vi "Critical.vi"(8 "error in (no error)":errorcluster, 9 "Source":string, 10 "Message":string, 11 "RQMHLogger in":refnum<class "RQMHLogger.lvclass">) -> (0 "error out":errorcluster, 3 "RQMHLogger out":refnum<class "RQMHLogger.lvclass">)   [LabVIEW 2024, in "RQMHLogger.lvclass"]
uses:
  RQMHLogger.lvclass
  RQMHLogger.lvclass/RQMHLogger.ctl
  Shared/Level.ctl
  Shared/LoggerShared.lvlib
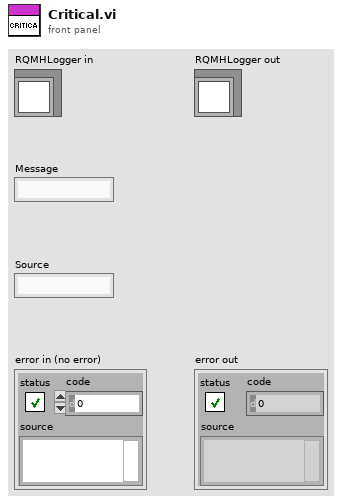
[diagram p1: front panel]
types:
  T1 = typedef "LoggerShared.lvlib/Level.ctl" = enum16{"DEBUG", "INFO", "WARNING", "ERROR", "CRITICAL"}
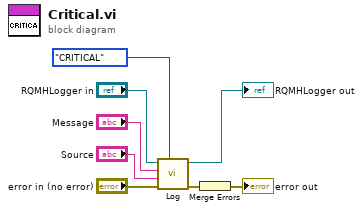
[diagram p0: block diagram]
diagram:
  n1 = call "Log.vi"("Level"=Level."CRITICAL", "Error to log"="error in (no error)", "Source"="Source", "Message"="Message", "RQMHLogger in"="RQMHLogger in") -> ("Errors"=w5:errorcluster[], "RQMHLogger out"=→"RQMHLogger out":refnum<class "RQMHLogger.lvclass">)  [unwired: 5 in]
  n2 = Merge Errors(w5) -> (→"error out":errorcluster)
